vi "Experiment Initialization.vi"(0 "Header Comments":string="This is a C(T) experiment being done in Physics 350.\r\nIt records the decay response of an RC circuit where the capacitance is a strong function of temperature.", 5 "Temperature Control Parameters":T3={"Start Temp"=40.0, "Temp Step"=10.0, "End Temp"=60.0} {"End Temp" format="%.2f"; "Temp Step" format="%.2f"; "Start Temp" format="%.2f"}, 9 "Timing Control Parameters":T2={"N cycles for averaging"=30, "N points per measurement"=1000, "Measurment time interval"=1e-05} {"Measurment time interval" format="%.2e"}, 11 "error in (no error)":errorcluster) -> (2 "Go Forward":bool, 3 "Auto Launch Data Viewer at End":bool=TRUE, 4 "data file path out":path, 6 "Temp Array":dbl[](array[numeric])=[40.0, 50.0, 60.0] format="%.2f", 8 "Timing Control Parameters out":T1={"N cycles for averaging"=100, "N points per measurment"=1000, "Measurment time interval"=1e-05} {"Measurment time interval" format="%.2e"}, 15 "error out":errorcluster)   [LabVIEW 2014]
doc: "This vi starts the C(T) expermental sequence. It creates the control parameters necessary for the rest of the experimental sequence. It allows for the option of loading the parameters from a pre-built template text file as well.\n\nPaul K Dixon\nPhysics 350\nCSUSB Physics"
uses:
  globals/C(T) global variables.vi
panel:
  in  "reload parameters":bool
  in  "default init data file name":string="P350 C(T) experimental data file"
  in  "exit":bool
  in  "go forward":bool
  out "File Header":string="This is a C(T) experiment being done in Physics 350.\r\nIt records the decay response of an RC circuit where the capacitance is a strong function of temperature.\r\n\r\n2/13/2004\r\n11:00 AM\r\n\r\nStart temp = 40.0\r\nTemp step = 10.0\r\nEnd temp = 60.0\r\nNum temps = 3\r\nNum avg cycles = 100\r\nNum points per meas = 1000\r\nMeas time interval = 1.00E-5\r\n\r\nDDD\r\n\r\n"
  out "N temps":i32=3
  in  "Auto Launch Data Viewer at End":bool=TRUE
  # "P350 C(T) Experimental Initialization"
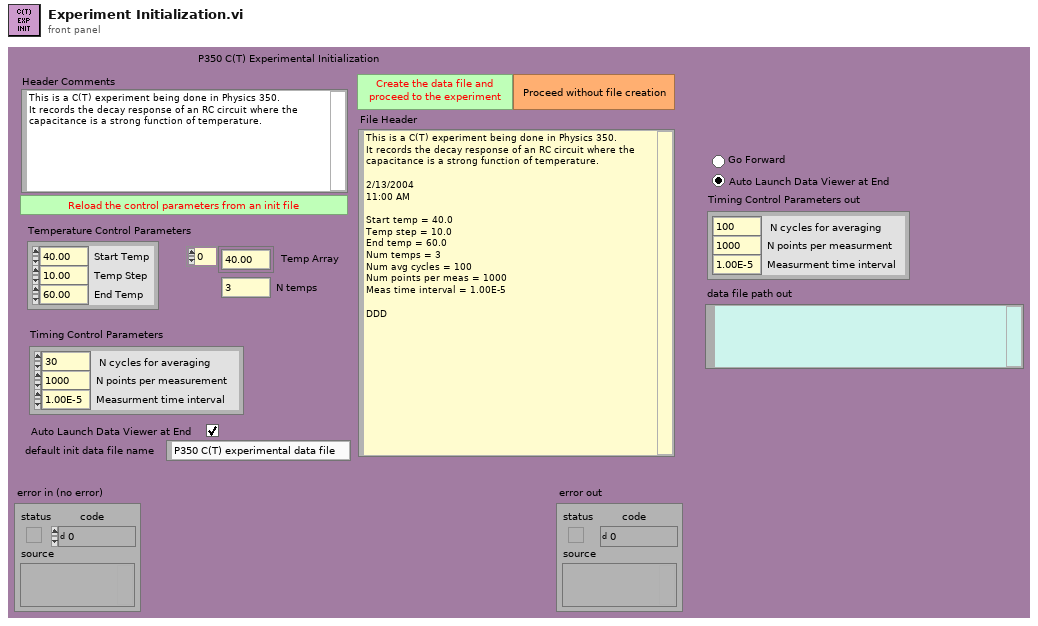
[diagram p1: front panel]
types:
  T1 = cluster{"N cycles for averaging":i32, "N points per measurment":i32, "Measurment time interval":dbl}
  T2 = cluster{"N cycles for averaging":i32, "N points per measurement":i32, "Measurment time interval":dbl}
  T3 = cluster{"Start Temp":dbl, "Temp Step":dbl, "End Temp":dbl}
  T4 = cluster{"Starting Value":dbl, "Step size":dbl, "Ending Value":dbl}
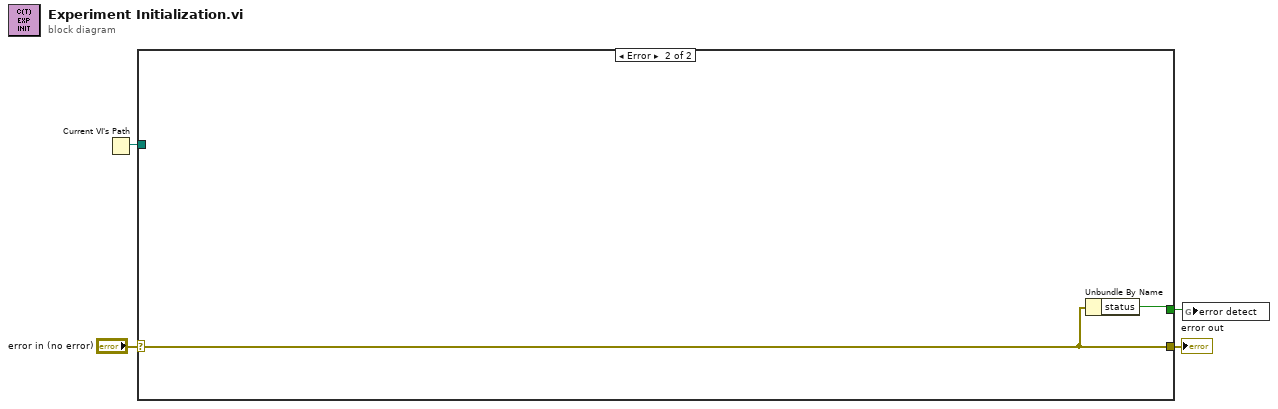
[diagram p0: block diagram]
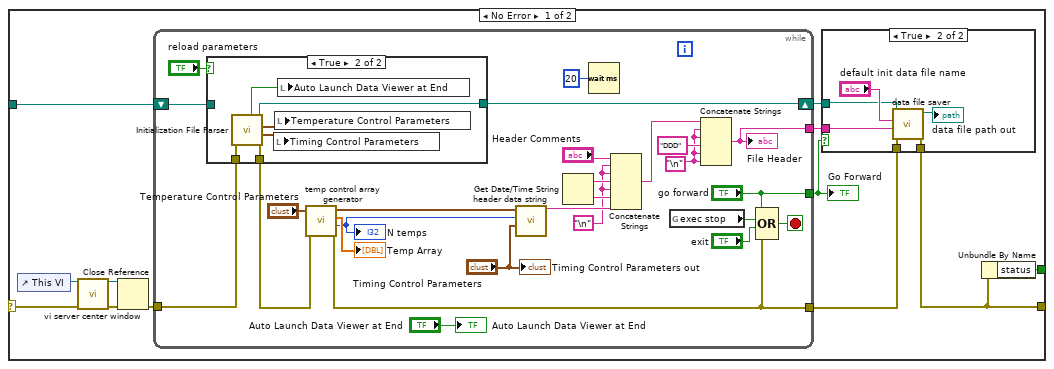
[diagram p2: hidden frame]
diagram:
  n1 = Current VI's Path() -> (path=w2:path)
  n2 = case shown="Error" "error in (no error)" {
    selector: "error in (no error)" -> [w10 w59]
    tunnel: [w6 w59] -> w4
    tunnel: w2 -> [w13 _]
    tunnel: [w5 w58] -> w1
    frame No Error {
      n3 = control-ref of="This VI"() -> (w11:refnum<vi>)
      n4 = call "vi server center window.vi"("VI ref in"=w11, "error in"=w10) -> ("VI ref out"=w7:refnum<vi>, "error out"=w9:errorcluster)  [unwired: 12 out]
      n5 = Close Reference(reference=w7, error in (no error)=w9) -> (error out=w8:errorcluster)
      n6 = while {
        shift-left: w13 -> [w24]
        shift-right: [w23] -> w12
        tunnel: ["go forward"] -> w15
        tunnel: [w42] -> w16
        tunnel: w8 -> [w18]
        tunnel: [w17] -> w14
        stop <- w21 stop-if-true
        w37 = "\n"
        w34 = "\n"
        n7 = case shown="True" "reload parameters" {
          tunnel: [w44 w48] -> w26
          tunnel: [w43 w47] -> w23
          tunnel: w18 -> [w44 w45]
          tunnel: w24 -> [w43 _]
          frame False {
          }
          frame True {
            n8 = call "Initialization File Parser.vi"("error in (no error)"=w45) -> ("error out"=w48:errorcluster, "Timing Control Parameters"=w49:T2, "Temperature Control Parameters"=w50:T3, "file path used"=w47:path, "Auto Launch Data Viewer at End"=w46:bool)  [unwired: 1 in, 5 out]
            n9 = local write "Timing Control Parameters"(w49) -> ()
            n10 = local write "Temperature Control Parameters"(w50) -> ()
            n11 = local write "Auto Launch Data Viewer at End"(w46) -> ()
          }
        }
        n12 = call "temp control array generator.vi"("error in (no error)"=w26, "T control in"="Temperature Control Parameters") -> ("error out"=w17:errorcluster, "N temps"=w30:i32, "Temp Values"=→"Temp Array":dbl[], "T control out"=w31:T4)  [unwired: 3 in, 3 out]
        "N temps" <- w30
        n13 = call "header data string.vi"("Timing Control Parameters"="Timing Control Parameters", "N temps"=w30, "Temperature Control Parameters"=w31) -> ("Concatenated String"=w41:string)  [unwired: 5 in, 3 out]
        n14 = Get Date/Time String() -> (date string=w40:string, time string=w39:string)  [unwired: 3 out]
        n15 = Wait (ms)(milliseconds to wait=u32 20) -> ()  [unwired: 1 out]
        n16 = Concatenate Strings("Header Comments", w34, w34, w40, w34, w39, w41) -> (w35:string)
        n17 = global read "C(T) global variables.vi" "exec stop"() -> (w20:bool)
        n18 = Concatenate Strings(w35, w37, w37, "DDD", w37, w37) -> (w42:string)
        "File Header" <- w42
        n19 = Compound Arithmetic op=OR("go forward", w20, "exit", w17) -> (w21:bool)
        "Auto Launch Data Viewer at End" <- "Auto Launch Data Viewer at End"
        "Timing Control Parameters out" <- "Timing Control Parameters"
      }
      "Go Forward" <- w15
      n20 = case shown="True" w15 {
        tunnel: w16 -> [_ w57]
        tunnel: w12 -> [_ w54]
        tunnel: w14 -> [w51 w53]
        tunnel: [w51 w52] -> w6
        frame False {
        }
        frame True {
          n21 = call "data file saver.vi"("error in (no error)"=w53, "Header String"=w57, "default data file name"="default init data file name", "reference file path in"=w54) -> ("error out"=w52:errorcluster, "data file path out"=→"data file path out":path)  [unwired: 6 out]
        }
      }
      n22 = Unbundle By Name(w6) -> ("status"=w5:bool)
    }
    frame Error {
      n23 = Unbundle By Name(w59) -> ("status"=w58:bool)
    }
  }
  "error out" <- w4
  n24 = global write "C(T) global variables.vi" "error detect"(w1) -> ()
